vi "数据模拟实测.vi"() -> ()   [LabVIEW 2020]
uses:
  <vilib>/Utility/error.llb/DialogType.ctl
  <vilib>/Analysis/baseanly.llb/Mean (DBL).vi
  <vilib>/Utility/inputDevices.llb/mouseAcquire.vi
  GlobalVariable.vi
  <vilib>/Analysis/NI_AALBase.lvlib
panel:
  in  "退出":bool
  in  "选项卡控件":enum32{"数据文件界面", "实时模拟界面"}(tab)
  out "历史波形图":dbl[][](graph)
  out "数据采集起止时间":string
  in  "曲线标尺":bool[](array[boolean])=[TRUE, TRUE, TRUE, TRUE, TRUE, TRUE, TRUE, TRUE]
  in  "曲线隐显":bool[](array[boolean])=[TRUE, TRUE, TRUE, TRUE, TRUE, TRUE, TRUE, TRUE]
  in  "开始模拟":bool
  in  "重选文件":bool
  in  "刻棒选择":u16(ring) items=["D棒位"]
  in  "因子选择":i32(ring) items=["C1", "C2", "C3", "C4", "C5", "C6", "C7", "C8", "C9", "10"]
  in  "上段信号选择":i32(ring) items=["电流1", "电流2"]
  in  "下段信号选择":u16(ring)=1 items=["电流1", "电流2"]
  out "实时波形图":sgl[][](graph) caption="Waveform Chart - Dark"
  in  "曲线开关0":bool
  in  "曲线开关1":bool
  in  "曲线开关2":bool
  in  "曲线开关3":bool
  in  "曲线开关5":bool
  in  "曲线开关4":bool
  in  "自动调整Y标尺？":bool
  in  "自动/手动调整X标尺？":bool
  out "曲线0数字":dbl caption="电流1"
  out "曲线1数字":dbl caption="电流1反应性"
  out "曲线2数字":dbl caption="电流2"
  out "曲线3数字":dbl caption="电流2反应性"
  out "曲线4数字":dbl caption="D棒位"
  out "曲线5数字":dbl
  in  "仿真加速或减速倍数":dbl(slide)=0.1 min=-5.0 max=10.0 step=0.1 scale=-5.0..10.0 scale format="%#.1f"
  in  "备注说明":string
  out "上下段比值":dbl format="%0.2f"
  in  "合并DSF":bool
  in  "DRWM启用":bool
  in  "上段本底":dbl
  in  "下段本底":dbl
  in  "X标尺最小+":bool
  in  "X标尺最小-":bool
  in  "Y标尺最小+":bool
  in  "Y标尺最小-":bool
  in  "Y标尺最大+":bool
  in  "Y标尺最大-":bool
  out "AllStop":bool
  # "DRWM选项"
  # "DRWM控制"
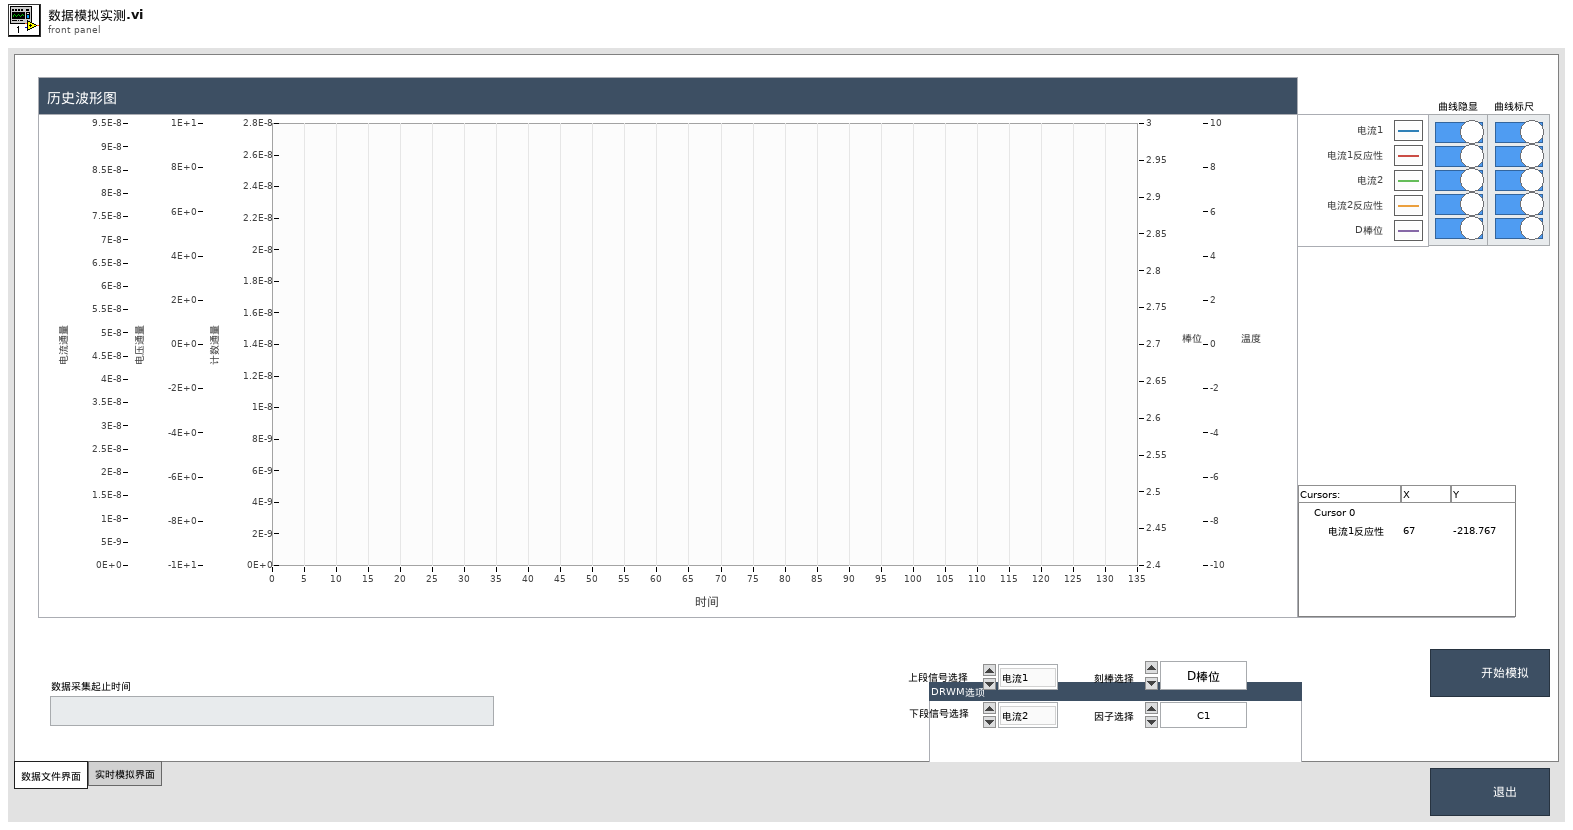
[diagram p1: front panel]
types:
  T1 = enum32{"Page Enabled", "Page Disabled", "Page Disabled & Grayed"}
  T2 = enum8{"Enabled", "Disabled", "Disabled and Grayed Out"}
  T3 = enum16{"open", "open or create", "create or replace", "create", "open (read only)"}
  T4 = typedef "DialogType.ctl" = u16
  T5 = cluster{"button 1":bool, "button 2":bool, "button 3":bool, "button 4":bool}
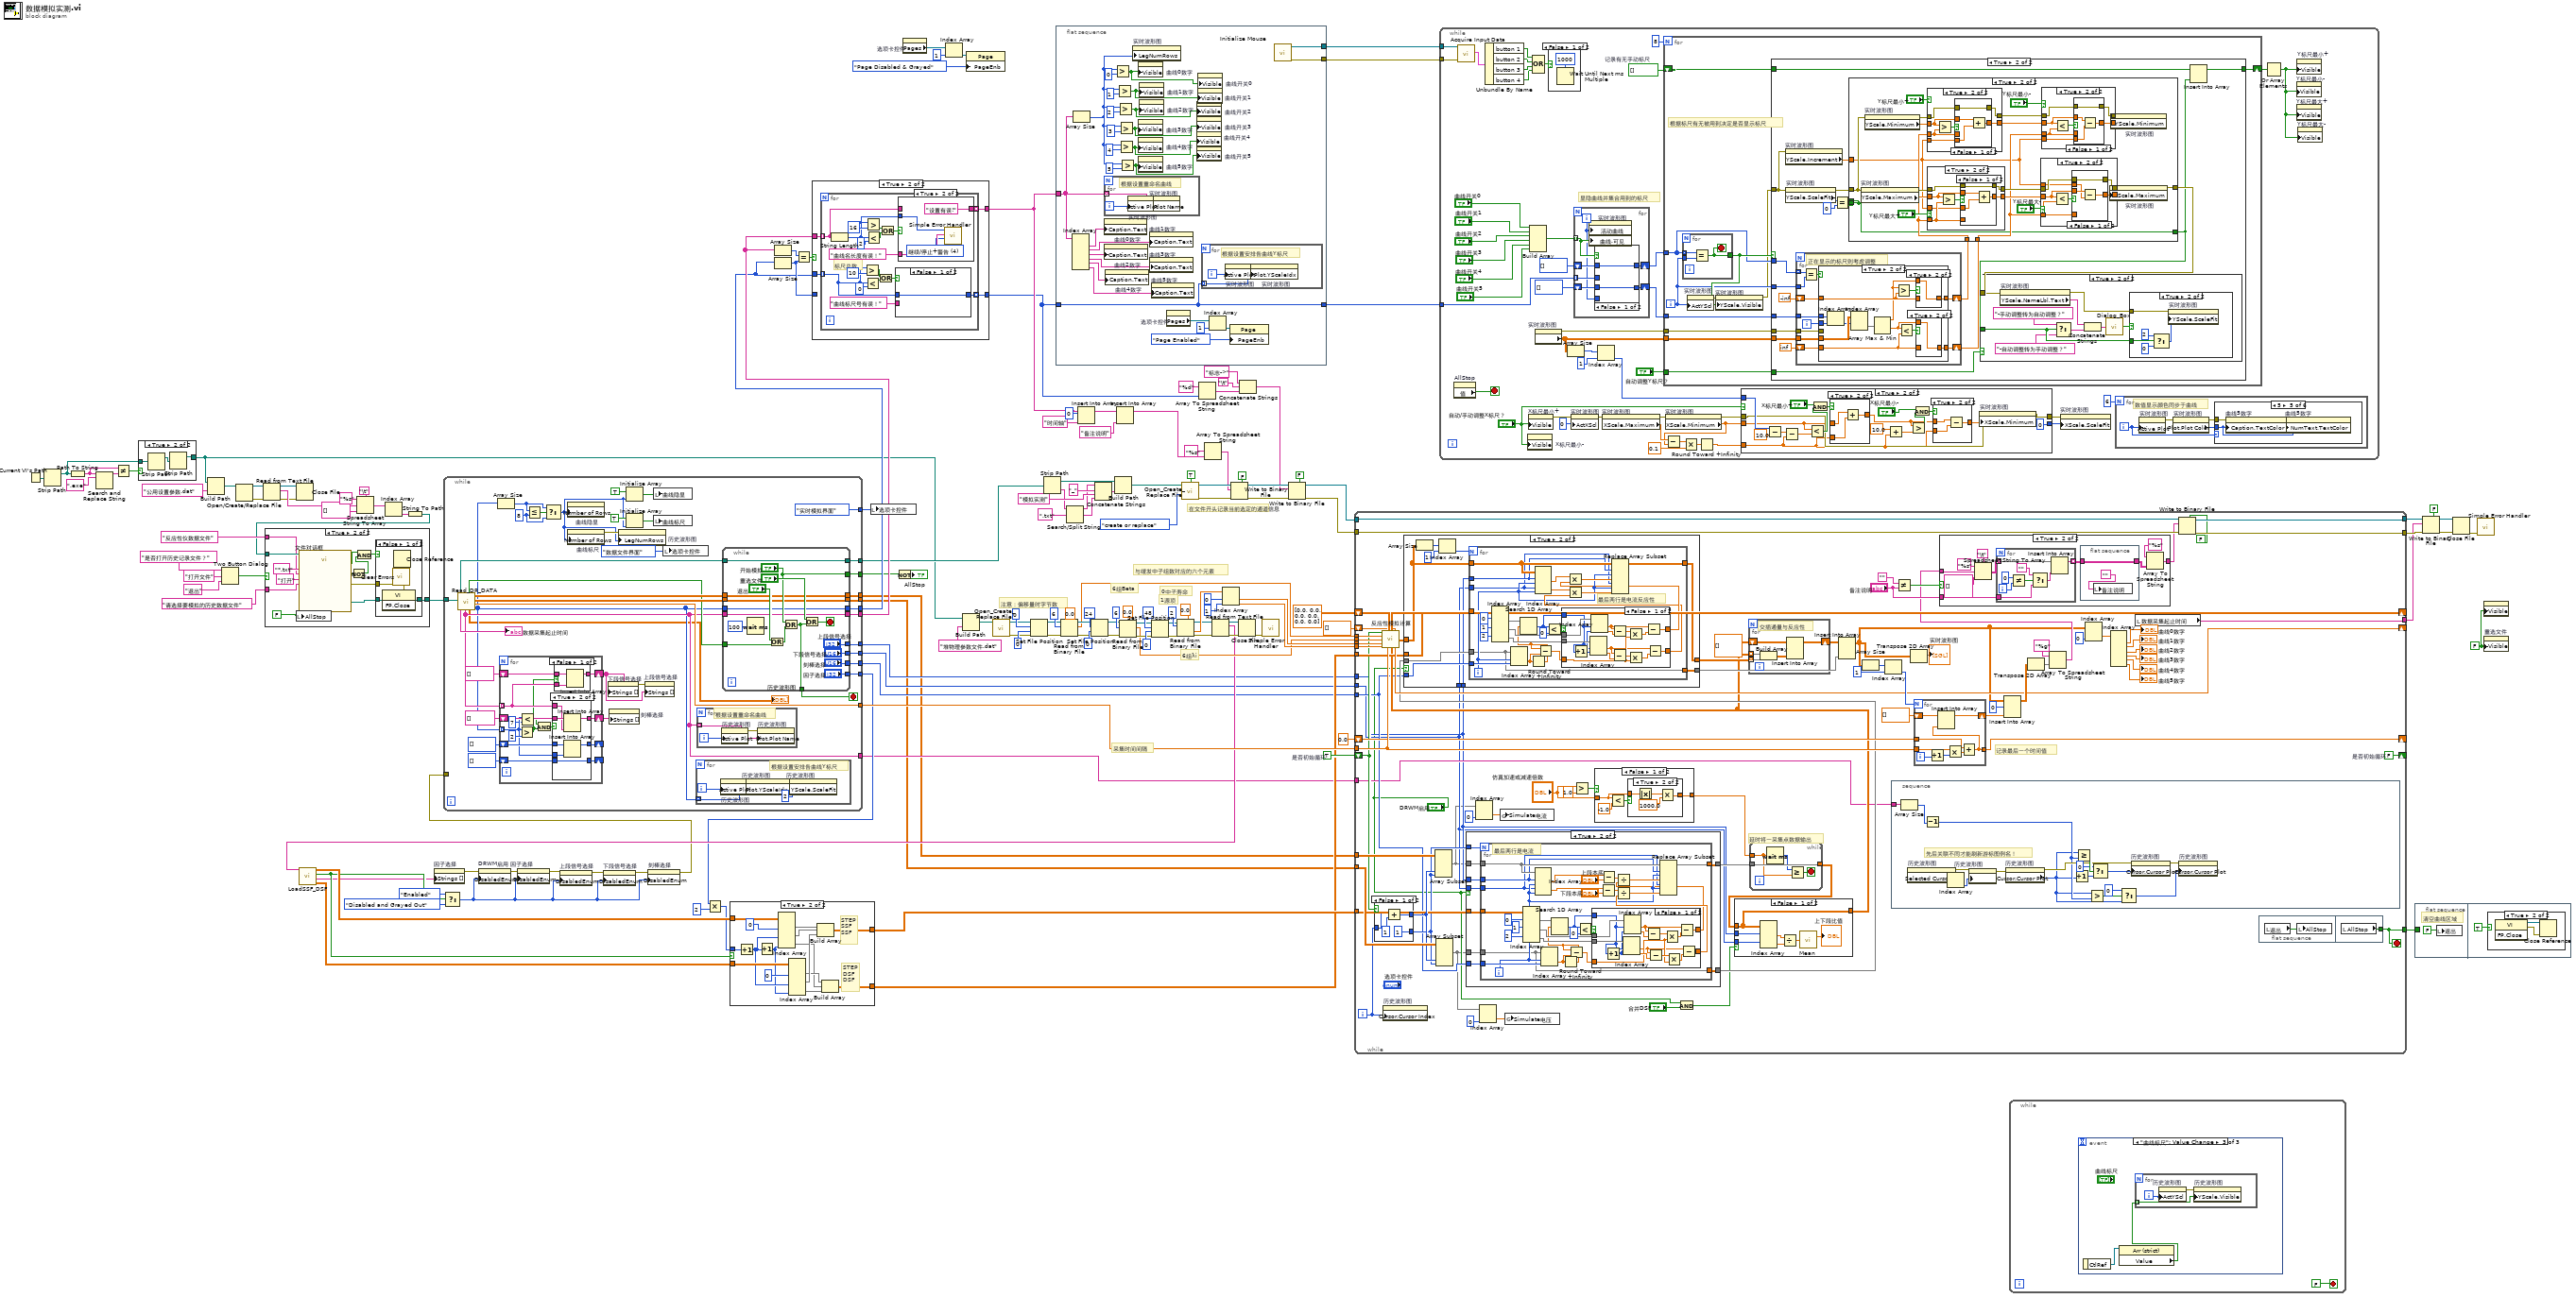
[diagram p0: block diagram]
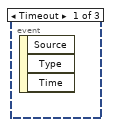
[diagram p2: hidden frame]
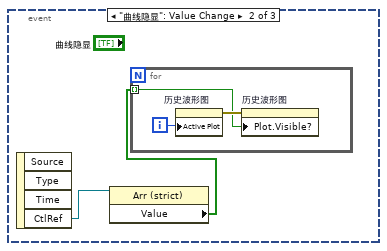
[diagram p3: hidden frame]
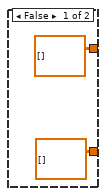
[diagram p4: hidden frame]
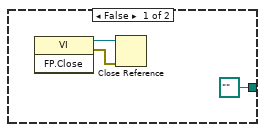
[diagram p5: hidden frame]
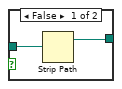
[diagram p7: hidden frame]
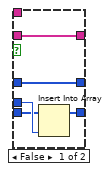
[diagram p9: hidden frame]
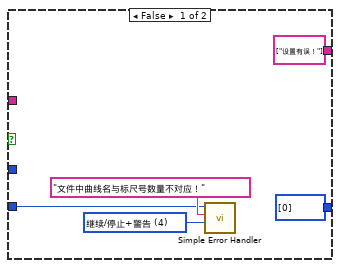
[diagram p11: hidden frame]
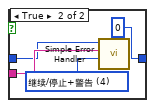
[diagram p12: hidden frame]
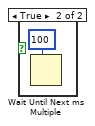
[diagram p14: hidden frame]
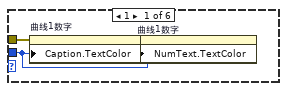
[diagram p15: hidden frame]
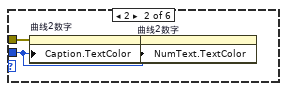
[diagram p16: hidden frame]
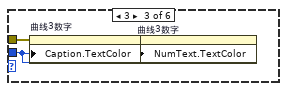
[diagram p17: hidden frame]
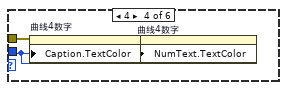
[diagram p18: hidden frame]
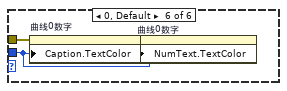
[diagram p19: hidden frame]
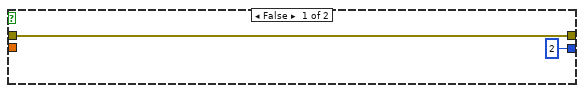
[diagram p20: hidden frame]
diagram:
  w5 = FALSE ("Visible")
  w122 = TRUE  # 是否初始循环
  # "6组λi"
  # "在文件开头记录当前选定的通道信息"
  # "采集时间间隔"
  # "注意：偏移量时字节数"
  # "与缓发中子组数对应的六个元素"
  # "0中子寿命"
  # "1源项"
  # "6组Beta"
  n1 = Current VI's Path() -> (path=w66:path)
  n2 = Strip Path(path=w66) -> (stripped path=w61:path)  [unwired: 1 out]
  n3 = Path To String(path=w61) -> (string=w63:string)
  n4 = Search and Replace String(input string=w63, search string=".exe" ("搜索字符串")) -> (result string=w64:string)  [unwired: 6 in, 3 out]
  n5 = Not Equal?(x=w63, y=w64) -> (x != y?=w62:bool)
  n6 = case shown="True" w62 {
    tunnel: w61 -> [w155 w158]
    tunnel: [w154 w156] -> w29
    frame False {
      n7 = Strip Path(path=w155) -> (stripped path=w154:path)  [unwired: 1 out]
    }
    frame True {
      n8 = Strip Path(path=w158) -> (stripped path=w157:path)  [unwired: 1 out]
      n9 = Strip Path(path=w157) -> (stripped path=w156:path)  [unwired: 1 out]
    }
  }
  n10 = Build Path(base path=w29, name or relative path="公用设置参数.dat") -> (appended path=w47:path)
  n11 = Two Button Dialog(message="是否打开历史记录文件？", 1:"退出" ("message"), 2:"打开文件" ("message")) -> (T button?=w57:bool)
  n12 = Open/Create/Replace File(file path (use dialog)=w47) -> (refnum out=w50:refnum<file>, error out=w51:errorcluster)  [unwired: 5 in, 1 out]
  n13 = Read from Text File(file (use dialog)=w50, error in=w51) -> (refnum out=w49:refnum<file>, text=w55:string, error out=w48:errorcluster)  [unwired: 1 in, 2 out]
  n14 = Close File(refnum=w49, error in=w48) -> ()  [unwired: 2 out]
  n15 = Spreadsheet String To Array(delimiter (Tab)="\t", format string="%s", spreadsheet string=w55, array type (2D Dbl)=string[] [] ("添加的数组")) -> (array=w56:string[])
  n16 = Index Array(array=w56) -> (element=w45:string)  [unwired: 1 in]
  n17 = String To Path(string=w45) -> (path=w58:path)
  n18 = case shown="True" w57 {
    tunnel: w58 -> [_ w174]
    tunnel: "请选择要模拟的历史数据文件" ("prompt") -> [_ w170]
    tunnel: "反应性仪数据文件" ("pattern label") -> [_ w169]
    tunnel: [path "" ("selected path") w167] -> w41
    frame False {
      n19 = invoke class="VI" method="FP.Close"() -> (reference out=w160:refnum<vi>, error out=w159:errorcluster)  [unwired: 3 in, 1 out]
      n20 = Close Reference(reference=w160, error in (no error)=w159) -> ()  [unwired: 1 out]
    }
    frame True {
      n21 = local write "AllStop"(FALSE ("退出程序")) -> ()
      n22 = call "文件对话框"("start path"=w174, "prompt"=w170, "button label"="打开", "pattern (all files)"="*.txt", "pattern label"=w169) -> ("selected path"=w168:path, "exists"=w165:bool, "cancelled"=w166:bool, "error out"=w162:errorcluster)  [unwired: 7 in]
      n23 = Not(x=w166) -> (.not. x?=w164:bool)
      n24 = And(x=w165, y=w164) -> (x .and. y?=w163:bool)
      n25 = case shown="False" w163 {
        tunnel: w168 -> [w178 w179]
        tunnel: [w178 w179] -> w167
        tunnel: w162 -> [w177 _]
        frame False {
          n26 = invoke class="VI" method="FP.Close"() -> (reference out=w175:refnum<vi>, error out=w176:errorcluster)  [unwired: 3 in, 1 out]
          n27 = call <vilib>:"Clear Errors.vi"("error in (no error)"=w177) -> ()  [unwired: 5 in, 2 out]
          n28 = Close Reference(reference=w175, error in (no error)=w176) -> ()  [unwired: 1 out]
        }
        frame True {
        }
      }
    }
  }
  n29 = property on="选项卡控件" class="TabCtl (strict)"() -> ("Pages"=w1:refnum<vi>[])  [unwired: 2 in, 2 out]
  n30 = Index Array(array=w1, index=1) -> (element=w2:refnum<vi>)
  n31 = Build Path(base path=w29, name or relative path="堆物理参数文件.dat" ("string")) -> (appended path=w134:path)
  n32 = property class="Page"(reference=w2, "PageEnb"=T1."Page Disabled & Grayed" ("Page Enabled State")) -> ()  [unwired: 1 in, 2 out]
  n33 = call <vilib>:"Open_Create_Replace File.vi"("file path"=w134) -> ("error out"=w118:errorcluster, "refnum"=w119:refnum<file>)  [unwired: 7 in, 2 out]
  n34 = Set File Position(offset (in bytes) (0)=0, refnum=w119, from (0:start)=0, error in=w118) -> (refnum out=w131:refnum<file>, error out=w130:errorcluster)
  n35 = flat-sequence {
    tunnel: w85 -> [w194]
    tunnel: [w184] -> w112
    tunnel: w84 -> [w184]
    tunnel: [w186] -> w121
    tunnel: [w185] -> w120
    frame #0 {
      n36 = Index Array(array=w194) -> (element #1=w206:string, element #2=w205:string, element #3=w204:string, element #4=w203:string, element #5=w202:string, element #6=w201:string)  [unwired: 6 in]
      n37 = Array Size(array=w194) -> (size(s)=w187:i32)
      n38 = property on="曲线0数字" class="DigNum (strict)"("Caption.Text"=w206) -> ()  [unwired: 2 in, 2 out]
      n39 = for {
        tunnel: w194 -> [w211] mode=indexing
        i -> [w212]
        # "根据设置重命名曲线"
        n40 = property on="实时波形图" class="WFChart (strict)"("Active Plot"=w212) -> (error out=w210:errorcluster)  [unwired: 2 in, 1 out]
        n41 = property on="实时波形图" class="WFChart (strict)"(error in=w210, "Plot.Plot Name"=w211) -> ()  [unwired: 1 in, 2 out]
      }
      n42 = property on="曲线2数字" class="DigNum (strict)"("Caption.Text"=w204) -> ()  [unwired: 2 in, 2 out]
      n43 = property on="曲线4数字" class="DigNum (strict)"("Caption.Text"=w202) -> ()  [unwired: 2 in, 2 out]
      n44 = Greater?(x=w187, y=0) -> (0:w193:bool)
      n45 = Greater?(x=w187, y=1) -> (0:w192:bool)
      n46 = Greater?(x=w187, y=2) -> (0:w191:bool)
      n47 = Greater?(x=w187, y=3) -> (0:w190:bool)
      n48 = Greater?(x=w187, y=4) -> (0:w189:bool)
      n49 = Greater?(x=w187, y=5) -> (0:w188:bool)
      n50 = property on="实时波形图" class="WFChart (strict)"("LegNumRows"=w187) -> ()  [unwired: 2 in, 2 out]
      n51 = property on="曲线0数字" class="DigNum (strict)"("Visible"=w193) -> ()  [unwired: 2 in, 2 out]
      n52 = property on="曲线3数字" class="DigNum (strict)"("Visible"=w190) -> ()  [unwired: 2 in, 2 out]
      n53 = property on="曲线4数字" class="DigNum (strict)"("Visible"=w189) -> ()  [unwired: 2 in, 2 out]
      n54 = property on="曲线5数字" class="DigNum (strict)"("Visible"=w188) -> ()  [unwired: 2 in, 2 out]
      n55 = property on="曲线1数字" class="DigNum (strict)"("Visible"=w192) -> ()  [unwired: 2 in, 2 out]
      n56 = property on="曲线2数字" class="DigNum (strict)"("Visible"=w191) -> ()  [unwired: 2 in, 2 out]
      n57 = property on="曲线1数字" class="DigNum (strict)"("Caption.Text"=w205) -> ()  [unwired: 2 in, 2 out]
      n58 = property on="曲线3数字" class="DigNum (strict)"("Caption.Text"=w203) -> ()  [unwired: 2 in, 2 out]
      n59 = property on="曲线5数字" class="DigNum (strict)"("Caption.Text"=w201) -> ()  [unwired: 2 in, 2 out]
      n60 = property on="选项卡控件" class="TabCtl (strict)"() -> ("Pages"=w183:refnum<vi>[])  [unwired: 2 in, 2 out]
      n61 = property on="曲线开关4" class="Bool (strict)"("Visible"=w189) -> ()  [unwired: 2 in, 2 out]
      n62 = property on="曲线开关2" class="Bool (strict)"("Visible"=w191) -> ()  [unwired: 2 in, 2 out]
      n63 = property on="曲线开关3" class="Bool (strict)"("Visible"=w190) -> ()  [unwired: 2 in, 2 out]
      n64 = property on="曲线开关5" class="Bool (strict)"("Visible"=w188) -> ()  [unwired: 2 in, 2 out]
      n65 = property on="曲线开关1" class="Bool (strict)"("Visible"=w192) -> ()  [unwired: 2 in, 2 out]
      n66 = property on="曲线开关0" class="Bool (strict)"("Visible"=w193) -> ()  [unwired: 2 in, 2 out]
      n67 = for {
        tunnel: w184 -> [w207] mode=indexing
        i -> [w209]
        # "根据设置安排各曲线Y标尺"
        n68 = property on="实时波形图" class="WFChart (strict)"("Active Plot"=w209) -> (error out=w208:errorcluster)  [unwired: 2 in, 1 out]
        n69 = property on="实时波形图" class="WFChart (strict)"(error in=w208, "Plot.YScaleIdx"=w207) -> ()  [unwired: 1 in, 2 out]
      }
      n70 = Index Array(array=w183, index=1) -> (element=w182:refnum<vi>)
      n71 = property class="Page"(reference=w182, "PageEnb"=T1."Page Enabled" ("Page Enabled State")) -> ()  [unwired: 1 in, 2 out]
      n72 = call <vilib>:"Initialize Mouse.vi"() -> ("error out"=w186:errorcluster, "device ID"=w185:refnum<k1>)  [unwired: 1 in, 9 out]
    }
  }
  n73 = Read from Binary File(5:sgl 0.0, 8:w130, 10:6, 11:w131) -> (0:w126:errorcluster, 2:w117:sgl[], 3:w127:refnum<file>)  [unwired: 2 in, 1 out]
  n74 = Set File Position(offset (in bytes) (0)=24, refnum=w127, from (0:start)=0, error in=w126) -> (refnum out=w129:refnum<file>, error out=w128:errorcluster)
  n75 = Read from Binary File(5:sgl 0.0, 8:w128, 10:6, 11:w129) -> (0:w124:errorcluster, 2:w75:sgl[], 3:w125:refnum<file>)  [unwired: 2 in, 1 out]
  n76 = Set File Position(offset (in bytes) (0)=48, refnum=w125, from (0:start)=0, error in=w124) -> (refnum out=w133:refnum<file>, error out=w132:errorcluster)
  n77 = Read from Binary File(5:sgl 0.0, 8:w132, 10:2, 11:w133) -> (0:w39:errorcluster, 2:w144:sgl[], 3:w40:refnum<file>)  [unwired: 2 in, 1 out]
  n78 = Read from Text File(file (use dialog)=w40, error in=w39) -> (refnum out=w38:refnum<file>, text=w36:string, error out=w37:errorcluster)  [unwired: 1 in, 2 out]
  n79 = call "LoadSSF_DSF.vi"("SF_PATH"=w36) -> ("下段因子数据"=w34:dbl[][], "因子棒号"=w25:string[], "SF_OK"=w28:bool, "上段因子数据"=w35:dbl[][])  [unwired: 6 in, 1 out]
  n80 = property on="因子选择" class="Ring (strict)"("Strings []"=w25) -> (error out=w24:errorcluster)  [unwired: 2 in, 1 out]
  n81 = Select(t=T2."Enabled" ("禁用"), s=w28, f=T2."Disabled and Grayed Out" ("禁用")) -> (s? t:f=w19:T2)
  n82 = property on="DRWM启用" class="Bool (strict)"(error in=w24, "DisabledEnum"=w19) -> (error out=w23:errorcluster)  [unwired: 1 in, 1 out]
  n83 = property on="因子选择" class="Ring (strict)"(error in=w23, "DisabledEnum"=w19) -> (error out=w21:errorcluster)  [unwired: 1 in, 1 out]
  n84 = property on="上段信号选择" class="Ring (strict)"(error in=w21, "DisabledEnum"=w19) -> (error out=w20:errorcluster)  [unwired: 1 in, 1 out]
  n85 = property on="下段信号选择" class="Ring (strict)"(error in=w20, "DisabledEnum"=w19) -> (error out=w18:errorcluster)  [unwired: 1 in, 1 out]
  n86 = property on="刻棒选择" class="Ring (strict)"(error in=w18, "DisabledEnum"=w19) -> (error out=w17:errorcluster)  [unwired: 1 in, 1 out]
  n87 = while {
    tunnel: [w249] -> w11
    tunnel: [w251] -> w69
    tunnel: [w250] -> w111
    tunnel: [w247] -> w110
    tunnel: [w248] -> w10
    tunnel: [w240] -> w108
    tunnel: [w245] -> w68
    tunnel: w41 -> [w244]
    tunnel: w17 -> [_]
    tunnel: [w237] -> w22
    tunnel: [w229] -> w14
    tunnel: [w228] -> w15
    tunnel: [w227] -> w16
    tunnel: [w226] -> w13
    tunnel: [enum32{"数据文件界面", "实时模拟界面"}."实时模拟界面" ("选项卡控件")] -> w12
    stop <- w246 stop-if-true
    w224 = 8 ("y")
    n88 = call "Read_DR_DATA.vi"("文件路径"=w244) -> ("标尺号"=w222:i32[], "时间步长"=w240:dbl, "P2数据"=w242:dbl[][], "通量数据"=w243:dbl[][], "曲线数据"=→"历史波形图":dbl[][], "读取正确?"=w241:bool, "曲线名称"=w226:string[], "数据采集起止时间"=→"数据采集起止时间":string, "filepath"=w239:path)  [unwired: 2 in]
    n89 = Array Size(array=w222) -> (size(s)=w223:i32)
    n90 = for {
      tunnel: w226 -> [w253] mode=indexing
      tunnel: w222 -> [w259] mode=indexing
      shift-right: [w265] -> w230
      shift-left: string[] [] -> [w266]
      shift-right: [w263] -> _
      shift-left: i32[] [] ("标尺号") -> [w264]
      shift-right: [w254] -> w231
      shift-left: string[] [] -> [w255]
      shift-right: [w261] -> _
      shift-left: i32[] [] ("标尺号") -> [w262]
      n91 = Greater?(x=w259, y=2) -> (0:w252:bool)
      n92 = Less?(x=w259, y=7) -> (x < y?=w257:bool)
      n93 = And(x=w257, y=w252) -> (x .and. y?=w256:bool)
      n94 = case shown="True" w256 {
        tunnel: w266 -> [w275 w282]
        tunnel: [w275 w281] -> w265
        tunnel: w264 -> [w274 w280]
        tunnel: [w274 w279] -> w263
        tunnel: w259 -> [w273 w278]
        tunnel: w253 -> [_ w277]
        tunnel: w262 -> [w272 w276]
        tunnel: [w271 w276] -> w261
        frame False {
          n95 = Insert Into Array(array=w272, new element=w273) -> (w271:i32[])  [unwired: 1 in]
        }
        frame True {
          n96 = Insert Into Array(array=w282, new element=w277) -> (w281:string[])  [unwired: 1 in]
          n97 = Insert Into Array(array=w280, new element=w278) -> (w279:i32[])  [unwired: 1 in]
        }
      }
      n98 = case shown="False" w252 {
        tunnel: w255 -> [w269 w270]
        tunnel: [w268 w270] -> w254
        tunnel: w253 -> [w267 _]
        frame False {
          n99 = Insert Into Array(array=w269, new element=w267) -> (w268:string[])  [unwired: 1 in]
        }
        frame True {
        }
      }
    }
    n100 = Less Or Equal?(x=w223, y=w224) -> (x <= y?=w225:bool)
    n101 = Select(t=w223, s=w225, f=w224) -> (s? t:f=w215:i32)
    n102 = property on="曲线隐显" class="Arr (strict)"("Number of Rows"=w215) -> ()  [unwired: 2 in, 2 out]
    n103 = property on="曲线标尺" class="Arr (strict)"("Number of Rows"=w215) -> (error out=w216:errorcluster)  [unwired: 2 in, 1 out]
    n104 = property on="下段信号选择" class="Ring (strict)"("Strings []"=w231) -> (error out=w232:errorcluster)  [unwired: 2 in, 1 out]
    n105 = property on="刻棒选择" class="Ring (strict)"("Strings []"=w230) -> ()  [unwired: 2 in, 2 out]
    n106 = property on="历史波形图" class="WFGraph (strict)"(error in=w216, "LegNumRows"=w215) -> ()  [unwired: 1 in, 2 out]
    n107 = Initialize Array(TRUE ("开始模拟"), w215) -> (w219:bool[])
    n108 = Initialize Array(TRUE ("开始模拟"), w215) -> (w218:bool[])
    n109 = property on="上段信号选择" class="Ring (strict)"(error in=w232, "Strings []"=w231) -> ()  [unwired: 1 in, 2 out]
    n110 = local write "曲线隐显"(w219) -> ()
    n111 = local write "曲线标尺"(w218) -> ()
    n112 = local write "选项卡控件"(enum32{"数据文件界面", "实时模拟界面"}."数据文件界面" ("选项卡控件")) -> ()
    n113 = for {
      tunnel: w222 -> [w285] mode=indexing
      i -> [w287]
      # "根据设置安排各曲线Y标尺"
      n114 = property on="历史波形图" class="WFGraph (strict)"("Active Plot"=w287) -> (error out=w286:errorcluster)  [unwired: 2 in, 1 out]
      n115 = property on="历史波形图" class="WFGraph (strict)"(error in=w286, "Plot.YScaleIdx"=w285) -> (error out=w284:errorcluster)  [unwired: 1 in, 1 out]
      n116 = property on="历史波形图" class="WFGraph (strict)"(error in=w284, "YScale.ScaleFit"=u8 2 ("Y标尺.标尺调节")) -> ()  [unwired: 1 in, 2 out]
    }
    n117 = for {
      tunnel: w226 -> [w289] mode=indexing
      i -> [w290]
      # "根据设置重命名曲线"
      n118 = property on="历史波形图" class="WFGraph (strict)"("Active Plot"=w290) -> (error out=w288:errorcluster)  [unwired: 2 in, 1 out]
      n119 = property on="历史波形图" class="WFGraph (strict)"(error in=w288, "Plot.Plot Name"=w289) -> ()  [unwired: 1 in, 2 out]
    }
    n120 = while {
      tunnel: [w299] -> w249
      tunnel: [w297] -> w250
      tunnel: w242 -> [w299]
      tunnel: w226 -> [w297]
      tunnel: [w305] -> w246
      tunnel: ["开始模拟"] -> w251
      tunnel: w241 -> [w302]
      tunnel: w243 -> [w300]
      tunnel: [w300] -> w248
      tunnel: w222 -> [w298]
      tunnel: [w298] -> w247
      tunnel: [w295] -> w245
      tunnel: w239 -> [w295]
      tunnel: ["因子选择"] -> w237
      tunnel: ["上段信号选择"] -> w229
      tunnel: ["下段信号选择"] -> w228
      tunnel: ["刻棒选择"] -> w227
      stop <- w296 stop-if-true
      n121 = Wait (ms)(milliseconds to wait=u32 100 ("等待时间（毫秒）")) -> ()  [unwired: 1 out]
      n122 = Or(x="退出", y=w302) -> (x .or. y?=w303:bool)
      n123 = Or(x="开始模拟", y=w303) -> (x .or. y?=w305:bool)
      n124 = Or(x="重选文件", y=w305) -> (x .or. y?=w296:bool)
    }
  }
  n125 = Multiply(x=w22, y=u16 2) -> (x*y=w32:i32)
  n126 = case shown="True" w28 {
    tunnel: w35 -> [_ w324]
    tunnel: w34 -> [_ w322]
    tunnel: w32 -> [_ w323]
    tunnel: [dbl[][] [] w315] -> w31
    tunnel: [dbl[][] [] w314] -> w30
    frame False {
    }
    frame True {
      # "STEP\nDSF\nDSF"
      # "STEP\nSSF\nSSF"
      n127 = Increment(x=w323) -> (x+1=w311:i32)
      n128 = Increment(x=w311) -> (x+1=w310:i32)
      n129 = Index Array(array=w324, index (col) #1=0 ("索引 (行)"), index (col) #2=w311, index (col) #3=w310) -> (element #1=w321:dbl[], element #2=w320:dbl[], element #3=w317:dbl[])  [unwired: 3 in]
      n130 = Index Array(array=w322, index (col) #1=0 ("索引 (行)"), index (col) #2=w311, index (col) #3=w310) -> (element #1=w318:dbl[], element #2=w319:dbl[], element #3=w316:dbl[])  [unwired: 3 in]
      n131 = Build Array(w321, w320, w319) -> (w315:dbl[][])
      n132 = Build Array(w318, w317, w316) -> (w314:dbl[][])
    }
  }
  n133 = Array Size(array=w111) -> (size(s)=w116:i32)
  n134 = Array Size(array=w110) -> (size(s)=w114:i32)
  n135 = Equal?(x=w116, y=w114) -> (x = y?=w115:bool)
  n136 = case shown="True" w115 {
    tunnel: w114 -> [w327 _]
    tunnel: w110 -> [_ w333]
    tunnel: w111 -> [_ w332]
    tunnel: [i32[] [0] w331] -> w84
    tunnel: [string[] ["设置有误！"] w330] -> w85
    frame False {
      w329 = T4 4 items=["无对话框", "确定信息", "继续或停止信息", "确定信息＋警告", "继续/停止+警告"] ("type of dialog (OK msg:1)")
      n137 = call <vilib>:"Simple Error Handler.vi"("error code (no error:0)"=w327, "error source (\" \")"="文件中曲线名与标尺号数量不对应！" ("error source (\" \")"), "type of dialog (OK msg:1)"=w329) -> ()  [unwired: 2 in, 5 out]
    }
    frame True {
      n138 = for {
        tunnel: w333 -> [w338] mode=indexing
        tunnel: w332 -> [w335] mode=indexing
        tunnel: [w336] -> w331 mode=indexing
        tunnel: [w334] -> w330 mode=indexing
        # "标尺总数"
        n139 = String Length(string=w335) -> (length=w340:i32)
        n140 = Greater?(x=w338, y=10) -> (0:w343:bool)
        n141 = Less?(x=w338, y=0) -> (x < y?=w342:bool)
        n142 = Greater?(x=w340, y=16) -> (0:w347:bool)
        n143 = Less?(x=w340, y=2) -> (x < y?=w348:bool)
        n144 = Or(x=w343, y=w342) -> (x .or. y?=w339:bool)
        n145 = Or(x=w347, y=w348) -> (x .or. y?=w346:bool)
        n146 = case shown="False" w339 {
          tunnel: "曲线标尺号有误！" ("error source (\" \")") -> [_ w355]
          tunnel: w338 -> [w351 w354]
          tunnel: [w351 0] -> w336
          frame False {
          }
          frame True {
            w353 = T4 4 items=["无对话框", "确定信息", "继续或停止信息", "确定信息＋警告", "继续/停止+警告"] ("type of dialog (OK msg:1)")
            n147 = call <vilib>:"Simple Error Handler.vi"("error code (no error:0)"=w354, "error source (\" \")"=w355, "type of dialog (OK msg:1)"=w353) -> ()  [unwired: 2 in, 5 out]
          }
        }
        n148 = case shown="True" w346 {
          tunnel: "曲线名长度有误！" ("error source (\" \")") -> [_ w360]
          tunnel: w340 -> [_ w359]
          tunnel: w335 -> [w356 _]
          tunnel: [w356 "设置有误!"] -> w334
          frame False {
          }
          frame True {
            w358 = T4 4 items=["无对话框", "确定信息", "继续或停止信息", "确定信息＋警告", "继续/停止+警告"] ("type of dialog (OK msg:1)")
            n149 = call <vilib>:"Simple Error Handler.vi"("error code (no error:0)"=w359, "error source (\" \")"=w360, "type of dialog (OK msg:1)"=w358) -> ()  [unwired: 2 in, 5 out]
          }
        }
      }
    }
  }
  n150 = local write "选项卡控件"(w12) -> ()
  n151 = Not(x=w69) -> (.not. x?=→"AllStop":bool)
  n152 = Strip Path(path=w68) -> (stripped path=w70:path, name=w9:string)
  n153 = Search/Split String(string=w9, search string/char (-)=".txt" ("搜索字符串/字符(-)")) -> (substring before match=w7:string, match + rest of string=w6:string)  [unwired: 1 in, 1 out]
  n154 = Insert Into Array(array=w85, index=0 ("索引"), new element="时间轴" ("新元素/子数组")) -> (w90:string[])
  n155 = Concatenate Strings ("连接字符串")(w7, "_" ("string"), "模拟实测" ("字符串"), w6) -> (w71:string)
  n156 = Build Path(base path=w70, name or relative path=w71) -> (appended path=w72:path)
  n157 = Insert Into Array(array=w90, new element="备注说明" ("新元素/子数组")) -> (w89:string[])  [unwired: 1 in]
  n158 = call <vilib>:"Open_Create_Replace File.vi"("advisory dialog? (display:T)"=TRUE, "function (open:0)"=T3."create or replace", "file path"=w72) -> ("error out"=w106:errorcluster, "refnum"=w103:refnum<file>)  [unwired: 5 in, 2 out]
  n159 = Array To Spreadsheet String(array=w84, 3:"%d" ("format string")) -> (spreadsheet string=w94:string)  [unwired: 1 in]
  n160 = Array To Spreadsheet String(array=w89, 3:"%s" ("format string")) -> (spreadsheet string=w101:string)  [unwired: 1 in]
  n161 = Index Array(array=w144, index #1=0, index #2=1) -> (element #1=w137:sgl, element #2=w136:sgl)
  n162 = Write to Binary File(file (use dialog)=w103, data=w101, error in=w106, 5:FALSE ("预置数组或字符串大小？(T)")) -> (refnum out=w96:refnum<file>, error out=w95:errorcluster)  [unwired: 2 in, 1 out]
  n163 = Close File(refnum=w38, error in=w37) -> (error out=w123:errorcluster)  [unwired: 1 out]
  n164 = Concatenate Strings("标志->" ("字符串"), "\t", w94) -> (w91:string)
  n165 = call <vilib>:"Simple Error Handler.vi"("error in (no error)"=w123) -> ()  [unwired: 4 in, 5 out]
  n166 = Write to Binary File(file (use dialog)=w96, data=w91, error in=w95, 5:FALSE ("预置数组或字符串大小？(T)")) -> (refnum out=w86:refnum<file>, error out=w87:errorcluster)  [unwired: 2 in, 1 out]
  n167 = while {
    shift-right: [w430] -> _
    shift-left: sgl[][] [[0.0], [0.0], [0.0], [0.0], [0.0], [0.0]] -> [w431]
    tunnel: w117 -> [w432]
    tunnel: w75 -> [w437]
    tunnel: w137 -> [w429]
    tunnel: w136 -> [w428]
    shift-right: [w436] -> _
    shift-left: w122 -> [w377]
    tunnel: w86 -> [w427]
    tunnel: w87 -> [w435]
    tunnel: [w361] -> w113
    tunnel: [w434] -> w79
    tunnel: w108 -> [w398]
    tunnel: [w426] -> w80
    tunnel: w10 -> [w410]
    tunnel: w11 -> [w409]
    tunnel: [w390] -> w74
    shift-right: [w395] -> _
    shift-left: 0.0 -> [w394]
    shift-right: [w391] -> _
    shift-left: sgl[] [] ("N(0)OUT") -> [w392]
    tunnel: w31 -> [w386]
    tunnel: w30 -> [w385]
    tunnel: w16 -> [w376]
    tunnel: w15 -> [w373]
    tunnel: w14 -> [w374]
    tunnel: w13 -> [w375]
    i -> [w378]
    stop <- w361 stop-if-true
    w436 = FALSE  # 是否初始循环
    # "记录最后一个时间值"
    # "延时将一采集点数据输出"
    n168 = case shown="False" w377 {
      tunnel: [w622 0 ("索引")] -> w407
      tunnel: [1 ("索引") 2 ("索引")] -> w383
      tunnel: w378 -> [w621 _]
      frame False {
        n169 = Add(x=w621, y=1) -> (x+y=w622:i32)
      }
      frame True {
      }
    }
    n170 = property on="历史波形图" class="WFGraph (strict)"("Cursor.Cursor Index"=w378) -> ()  [unwired: 2 in, 2 out]
    n171 = Array Subset(array=w410, index (col)=w407, length (col)=w383) -> (w369:dbl[][])  [unwired: 2 in]
    n172 = Array Subset(array=w409, index (col)=w407, length (col)=w383) -> (w368:dbl[][])  [unwired: 2 in]
    n173 = case shown="True" "DRWM启用" {
      tunnel: w369 -> [w530 w537]
      tunnel: [w530 w536] -> w389
      tunnel: w368 -> [w529 w539]
      tunnel: w386 -> [_ w538]
      tunnel: w383 -> [_ w535]
      tunnel: w376 -> [_ w534]
      tunnel: [w529 w533] -> w381
      tunnel: w374 -> [_ w532]
      tunnel: w373 -> [_ w531]
      frame False {
      }
      frame True {
        n174 = for {
          N: w535 -> [_]
          tunnel: w539 -> [w556]
          tunnel: w538 -> [w569]
          tunnel: w537 -> [w554]
          tunnel: [w558] -> w536
          tunnel: w534 -> [w568]
          tunnel: [w556] -> w533
          tunnel: w532 -> [w550]
          tunnel: w531 -> [w549]
          i -> [w557]
          # "最后两行是电流"
          n175 = Index Array(array=w569, index (row) #1=0 ("禁用的索引 (列)"), index (row) #2=1 ("索引 (列)"), index (row) #3=2 ("索引 (列)")) -> (element #1=w567:dbl[], element #2=w563:dbl[], element #3=w562:dbl[])  [unwired: 3 in]
          n176 = Index Array(array=w554, index (row) #1=w550, index (col) #1=w557, index (row) #2=w549, index (col) #2=w557) -> (element #1=w544:dbl, element #2=w542:dbl)
          n177 = Index Array(array=w556, index (row)=w557, index (col)=w568) -> (element=w553:dbl)
          n178 = Round Toward +Infinity(x=w553) -> (ceil(x): smallest int >= x=w552:dbl)
          n179 = Search 1D Array ("搜索一维数组")(1D array=w567, element=w552) -> (index of element=w564:i32)  [unwired: 1 in]
          n180 = Subtract(x=w552, y=w553) -> (x-y=w551:dbl)
          n181 = Less?(x=w564, y=0) -> (x < y?=w565:bool)
          n182 = case shown="False" w565 {
            tunnel: w564 -> [w582 _]
            tunnel: w563 -> [w584 _]
            tunnel: w562 -> [w583 _]
            tunnel: [w576 1.0] -> w555
            tunnel: [w572 1.0] -> w561
            tunnel: w551 -> [w573 _]
            frame False {
              n183 = Increment(x=w582) -> (x+1=w581:i32)
              n184 = Index Array(array=w583, index #1=w582, index #2=w581) -> (element #1=w570:dbl, element #2=w575:dbl)
              n185 = Index Array(array=w584, index #1=w582, index #2=w581) -> (element #1=w578:dbl, element #2=w580:dbl)
              n186 = Subtract(x=w578, y=w580) -> (x-y=w579:dbl)
              n187 = Subtract(x=w570, y=w575) -> (x-y=w574:dbl)
              n188 = Multiply(x=w579, y=w573) -> (x*y=w577:dbl)
              n189 = Multiply(x=w574, y=w573) -> (x*y=w571:dbl)
              n190 = Subtract(x=w578, y=w577) -> (x-y=w576:dbl)
              n191 = Subtract(x=w570, y=w571) -> (x-y=w572:dbl)
            }
            frame True {
              n192 = One Button Dialog(message="SSF文件棒位索引错误！" ("消息")) -> (true=w588:bool)  [unwired: 1 in]
              n193 = Stop(stop? (T)=w588) -> ()
            }
          }
          n194 = Subtract(x=w542, y="下段本底") -> (x-y=w543:dbl)
          n195 = Subtract(x=w544, y="上段本底") -> (x-y=w545:dbl)
          n196 = Divide(x=w545, y=w555) -> (x/y=w560:dbl)
          n197 = Divide(x=w543, y=w561) -> (x/y=w559:dbl)
          n198 = Replace Array Subset(array=w554, new element #1=w560, index (row) #1=w550, index (col) #1=w557, new element #2=w559, index (row) #2=w549, index (col) #2=w557) -> (w558:dbl[][])
        }
      }
    }
    n199 = Index Array(array=w369, index (col)=0 ("索引 (行)")) -> (element=w366:dbl[])  [unwired: 1 in]
    n200 = Index Array(array=w368, index (col)=0 ("索引 (行)")) -> (element=w367:dbl[])  [unwired: 1 in]
    n201 = global write "GlobalVariable.vi" "Simulate电流"(w366) -> ()
    n202 = global write "GlobalVariable.vi" "Simulate电压"(w367) -> ()
    n203 = Greater?(x="仿真加速或减速倍数", y=1.0) -> (0:w414:bool)
    n204 = case shown="False" w414 {
      tunnel: "仿真加速或减速倍数" -> [w626 w636]
      tunnel: [w627 w635] -> w412
      frame False {
        n205 = Less?(x=w626, y=-1.0) -> (x < y?=w628:bool)
        n206 = case shown="True" w628 {
          tunnel: [1000.0 w633] -> w627
          tunnel: w626 -> [_ w631]
          frame False {
          }
          frame True {
            n207 = Absolute Value(x=w631) -> (abs(x)=w632:dbl)
            n208 = Multiply(x=w632, y=1000.0) -> (x*y=w633:dbl)
          }
        }
      }
      frame True {
        n209 = Divide(x=u32 1000, y=w636) -> (x/y=w635:dbl)
      }
    }
    n210 = And(x="DRWM启用", y="合并DSF") -> (x .and. y?=w371:bool)
    n211 = while {
      tunnel: w389 -> [w641]
      tunnel: [w641] -> w380
      tunnel: w412 -> [w639]
      stop <- w638 stop-if-true
      n212 = Wait (ms)(milliseconds to wait=w639) -> (millisecond timer value=w640:u32)
      n213 = Greater Or Equal?(x=w640, y=w639) -> (x >= y?=w638:bool)
    }
    n214 = case shown="False" w371 {
      tunnel: w380 -> [w457 w470]
      tunnel: [w457 w469] -> w379
      tunnel: w374 -> [w456 w462]
      tunnel: w373 -> [w455 w463]
      frame False {
        n215 = Index Array(array=w457, index (row) #1=w456, index (row) #2=w455) -> (element #1=w461:dbl[], element #2=w460:dbl[])  [unwired: 2 in]
        n216 = Divide(x=w461, y=w460) -> (x/y=w459:dbl[])
        n217 = call-poly <vilib>:"Mean.vi"("X"=w459) -> ("mean"=→"上下段比值":dbl)  [unwired: 1 out]
      }
      frame True {
        n218 = local read "上下段比值"() -> (w467:dbl)
        n219 = Index Array(array=w470, index (row) #1=w462, index (row) #2=w463) -> (element #1=w468:dbl[], element #2=w465:dbl[])  [unwired: 2 in]
        n220 = Divide(x=w468, y=w467) -> (x/y=w466:dbl[])
        n221 = Add(x=w466, y=w465) -> (x+y=w464:dbl[])
        n222 = Replace Array Subset(array=w470, new element #1=w464, index (row) #1=w462, new element #2=w464, index (row) #2=w463) -> (w469:dbl[][])  [unwired: 2 in]
      }
    }
    n223 = call "反应性模拟计算.vi"("循环次数"=w377, "λi*Ci(0)"=w431, "N(0)IN"=w392, "βi"=w432, "λi"=w437, "中子寿命"=w429, "源项"=w428, "采集间隔"=w398, "中子注量率"=w379) -> ("λi*Ci(t)"=w430:sgl[][], "反应性OUT"=w388:sgl[][], "N(0)OUT"=w391:sgl[])  [unwired: 4 in]
    n224 = case shown="True" "DRWM启用" {
      tunnel: w388 -> [w472 w478]
      tunnel: [w472 w481] -> w387
      tunnel: w385 -> [_ w482]
      tunnel: w376 -> [_ w483]
      tunnel: w381 -> [w471 w480]
      tunnel: [w471 w479] -> w384
      tunnel: w374 -> [_ w474]
      tunnel: w373 -> [_ w473]
      frame False {
      }
      frame True {
        n225 = Array Size(array=w478) -> (size(s)=w477:i32[])
        n226 = Index Array(array=w477, index=1 ("索引")) -> (element=w475:i32)
        n227 = for {
          N: w475 -> [_]
          tunnel: w480 -> [w492]
          tunnel: w482 -> [w509]
          tunnel: w478 -> [w497]
          tunnel: [w494] -> w481
          tunnel: w483 -> [w508]
          tunnel: [w492] -> w479
          tunnel: w474 -> [w488]
          tunnel: w473 -> [w487]
          i -> [w493]
          # "最后两行是电流反应性"
          n228 = Index Array(array=w509, index (row) #1=0 ("禁用的索引 (列)"), index (row) #2=1 ("索引 (列)"), index (row) #3=2 ("索引 (列)")) -> (element #1=w507:dbl[], element #2=w503:dbl[], element #3=w502:dbl[])  [unwired: 3 in]
          n229 = Index Array(array=w492, index (row)=w493, index (col)=w508) -> (element=w490:dbl)
          n230 = Round Toward +Infinity(x=w490) -> (ceil(x): smallest int >= x=w491:dbl)
          n231 = Search 1D Array(1D array=w507, element=w491) -> (index of element=w504:i32)  [unwired: 1 in]
          n232 = Index Array(array=w497, index (row) #1=w488, index (col) #1=w493, index (row) #2=w487, index (col) #2=w493) -> (element #1=w501:sgl, element #2=w500:sgl)
          n233 = Subtract(x=w491, y=w490) -> (x-y=w489:dbl)
          n234 = Less?(x=w504, y=0) -> (x < y?=w505:bool)
          n235 = case shown="False" w505 {
            tunnel: w504 -> [w521 _]
            tunnel: w503 -> [w524 _]
            tunnel: w502 -> [w523 _]
            tunnel: [w511 1.0] -> w499
            tunnel: [w510 1.0] -> w498
            tunnel: w489 -> [w516 _]
            frame False {
              n236 = Increment(x=w521) -> (x+1=w522:i32)
              n237 = Index Array(array=w523, index #1=w521, index #2=w522) -> (element #1=w513:dbl, element #2=w519:dbl)
              n238 = Index Array(array=w524, index #1=w521, index #2=w522) -> (element #1=w514:dbl, element #2=w520:dbl)
              n239 = Subtract(x=w514, y=w520) -> (x-y=w518:dbl)
              n240 = Subtract(x=w513, y=w519) -> (x-y=w517:dbl)
              n241 = Multiply(x=w518, y=w516) -> (x*y=w515:dbl)
              n242 = Multiply(x=w517, y=w516) -> (x*y=w512:dbl)
              n243 = Subtract(x=w514, y=w515) -> (x-y=w511:dbl)
              n244 = Subtract(x=w513, y=w512) -> (x-y=w510:dbl)
            }
            frame True {
              n245 = One Button Dialog(message="SSF文件棒位索引错误！" ("消息")) -> (true=w528:bool)  [unwired: 1 in]
              n246 = Stop(stop? (T)=w528) -> ()
            }
          }
          n247 = Multiply(x=w501, y=w499) -> (x*y=w496:dbl)
          n248 = Multiply(x=w500, y=w498) -> (x*y=w495:dbl)
          n249 = Replace Array Subset(array=w497, new element #1=w496, index (row) #1=w488, index (col) #1=w493, new element #2=w495, index (row) #2=w487, index (col) #2=w493) -> (w494:sgl[][])
        }
      }
    }
    n250 = for {
      tunnel: w379 -> [w644] mode=indexing
      tunnel: w387 -> [w643] mode=indexing
      shift-right: [w645] -> w408
      shift-left: sgl[][] [] ("平滑掉数据") -> [w646]
      # "交插通量与反应性"
      n251 = Build Array(w644, w643) -> (w642:dbl[][])
      n252 = Insert Into Array(array=w646, new element=w642) -> (w645:sgl[][])  [unwired: 2 in]
    }
    n253 = Insert Into Array(array=w408, new element=w384) -> (w362:sgl[][])  [unwired: 2 in]
    n254 = Array Size(array=w362) -> (size(s)=w402:i32[])
    n255 = Index Array(array=w402, index=1 ("索引")) -> (element=w400:i32)
    n256 = stacked-sequence {
      tunnel: w375 -> [w447]
      frame #0 {
        # "先后关联不同才能刷新游标图例名！"
        n257 = Array Size(array=w447) -> (size(s)=w446:i32)
        n258 = property on="历史波形图" class="WFGraph (strict)"() -> (error out=w452:errorcluster, "Selected Cursors"=w454:u32[])  [unwired: 2 in, 1 out]
        n259 = Decrement(x=w446) -> (x-1=w441:i32)
        n260 = Index Array(array=w454) -> (element=w453:u32)  [unwired: 1 in]
        n261 = property on="历史波形图" class="WFGraph (strict)"(error in=w452, "Active Cursor"=w453) -> (error out=w451:errorcluster)  [unwired: 1 in, 1 out]
        n262 = property on="历史波形图" class="WFGraph (strict)"(error in=w451) -> (error out=w448:errorcluster, "Cursor.Cursor Plot"=w439:i32)  [unwired: 1 in, 1 out]
        n263 = Increment(x=w439) -> (x+1=w443:i32)
        n264 = Greater Or Equal?(x=w439, y=w441) -> (x >= y?=w450:bool)
        n265 = Greater?(x=w439, y=w441) -> (0:w442:bool)
        n266 = Select(t=0, s=w450, f=w443) -> (s? t:f=w445:i32)
        n267 = Select(t=0, s=w442, f=w439) -> (s? t:f=w440:i32)
        n268 = property on="历史波形图" class="WFGraph (strict)"(error in=w448, "Cursor.Cursor Plot"=w445) -> (error out=w449:errorcluster)  [unwired: 1 in, 1 out]
        n269 = property on="历史波形图" class="WFGraph (strict)"(error in=w449, "Cursor.Cursor Plot"=w440) -> ()  [unwired: 1 in, 2 out]
      }
    }
    n270 = Not Equal?(x="", y="备注说明") -> (x != y?=w406:bool)
    n271 = Transpose 2D Array(2D array=w362) -> (transposed array=→"实时波形图":sgl[][])
    n272 = for {
      N: w400 -> [_]
      tunnel: w394 -> [w594]
      tunnel: w398 -> [w596]
      shift-right: [w592] -> w397
      shift-left: sgl[] [] -> [w593]
      tunnel: [w591] -> w395
      i -> [w590]
      n273 = Increment(x=w590) -> (x+1=w589:i32)
      n274 = Multiply(x=w596, y=w589) -> (x*y=w595:dbl)
      n275 = Add(x=w594, y=w595) -> (x+y=w591:dbl)
      n276 = Insert Into Array(array=w593, new element=w591) -> (w592:sgl[])  [unwired: 1 in]
    }
    n277 = Insert Into Array ("数组插入")(array=w362, index (row)=0 ("索引 (行)"), new element=w397) -> (w396:sgl[][])  [unwired: 1 in]
    n278 = Transpose 2D Array(2D array=w396) -> (transposed array=w424:sgl[][])
    n279 = Array To Spreadsheet String(array=w424, 3:"%g" ("format string")) -> (spreadsheet string=w382:string)  [unwired: 1 in]
    n280 = case shown="True" w406 {
      tunnel: [w597 w598] -> w403
      tunnel: "备注说明" -> [_ w607]
      tunnel: w382 -> [w597 w602]
      frame False {
      }
      frame True {
        n281 = Spreadsheet String To Array(delimiter (Tab)="\t", format string="%s", spreadsheet string=w602, array type (2D Dbl)=string[][] [] ("添加的数组")) -> (array=w603:string[][])
        n282 = for {
          tunnel: w603 -> [w617] mode=indexing
          tunnel: [w616] -> w601 mode=indexing
          tunnel: w607 -> [w611]
          i -> [w615]
          n283 = Not Equal?(x=0 ("y"), y=w615) -> (x != y?=w613:bool)
          n284 = Select(t="", s=w613, f=w611) -> (s? t:f=w612:string)
          n285 = Insert Into Array(array=w617, new element=w612) -> (w616:string[])  [unwired: 1 in]
        }
        n286 = flat-sequence {
          tunnel: w601 -> [w608]
          tunnel: [w608] -> w599
          frame #0 {
            n287 = local write "备注说明"("") -> ()
          }
        }
        n288 = Array To Spreadsheet String(array=w599, 3:"%s" ("format string")) -> (spreadsheet string=w598:string)  [unwired: 1 in]
      }
    }
    n289 = Index Array(array=w362, index (col)=0 ("索引 (行)")) -> (element=w421:sgl[])  [unwired: 1 in]
    n290 = Index Array(array=w421) -> (element #1=→"曲线0数字":sgl, element #2=→"曲线1数字":sgl, element #3=→"曲线2数字":sgl, element #4=→"曲线3数字":sgl, element #5=→"曲线4数字":sgl, element #6=→"曲线5数字":sgl)  [unwired: 6 in]
    n291 = local read "数据采集起止时间"() -> (w390:string)
    n292 = Write to Binary File(file (use dialog)=w427, data=w403, error in=w435, 5:FALSE ("预置数组或字符串大小？(T)")) -> (refnum out=w426:refnum<file>, error out=w434:errorcluster)  [unwired: 2 in, 1 out]
    n293 = flat-sequence {
      tunnel: [w619] -> w361
      frame #0 {
        n294 = local read "退出"() -> (w618:bool)
        n295 = local write "AllStop"(w618) -> ()
      }
      frame #1 {
        n296 = local read "AllStop"() -> (w619:bool)
      }
    }
  }
  n297 = while {
    tunnel: w112 -> [w678]
    tunnel: w121 -> [w653]
    tunnel: w120 -> [w652]
    stop <- w692 stop-if-true
    w676 = bool[] []  # 记录有无手动标尺
    # "显隐曲线并集合用到的标尺"
    n298 = property on="AllStop" class="Bool (strict)"() -> ("值"=w692:bool)  [unwired: 2 in, 2 out]
    n299 = call-poly <vilib>:"Acquire Input Data.vi"("device ID"=w652, "error in (no error)"=w653) -> ("button info"=w654:T5)  [unwired: 1 in, 16 out]
    n300 = Unbundle By Name(w654) -> ("button 1"=w651:bool, "button 2"=w650:bool, "button 3"=w649:bool, "button 4"=w648:bool)
    n301 = property on="X标尺最小-" class="Bool"("Visible"="自动/手动调整X标尺？") -> ()  [unwired: 2 in, 2 out]
    n302 = property on="X标尺最小+" class="Bool"("Visible"="自动/手动调整X标尺？") -> (error out=w670:errorcluster)  [unwired: 2 in, 1 out]
    n303 = Build Array("曲线开关0", "曲线开关1", "曲线开关2", "曲线开关3", "曲线开关4", "曲线开关5") -> (w685:bool[])
    n304 = Compound Arithmetic op=OR(w651, w650, w649, w648) -> (w647:bool)
    n305 = property on="实时波形图" class="WFChart (strict)"() -> (error out=w679:errorcluster, "History Data"=w668:sgl[][])  [unwired: 2 in, 1 out]
    n306 = case shown="False" w647 {
      frame False {
        n307 = Wait Until Next ms Multiple(millisecond multiple=u32 1000) -> ()  [unwired: 1 out]
      }
      frame True {
        n308 = Wait Until Next ms Multiple(millisecond multiple=u32 100) -> ()  [unwired: 1 out]
      }
    }
    n309 = Array Size(array=w668) -> (size(s)=w667:i32[])
    n310 = property on="实时波形图" class="WFChart (strict)"(error in=w670, "ActXScl"=0 ("活动X标尺")) -> (error out=w664:errorcluster)  [unwired: 1 in, 1 out]
    n311 = for {
      tunnel: w685 -> [w915] mode=indexing
      tunnel: w678 -> [w913] mode=indexing
      shift-right: [w912] -> w682
      shift-left: i32[] [] ("添加的数组") -> [w914]
      shift-right: [w909] -> w680
      shift-left: i32[] [] ("添加的数组") -> [w911]
      i -> [w910]
      n312 = property on="实时波形图" class="WFChart (strict)"("活动曲线"=w910, "曲线.可见"=w915) -> ()  [unwired: 2 in, 2 out]
      n313 = case shown="False" w915 {
        tunnel: w914 -> [w917 w923]
        tunnel: w913 -> [_ w922]
        tunnel: [w917 w921] -> w912
        tunnel: w911 -> [w916 w920]
        tunnel: w910 -> [_ w919]
        tunnel: [w916 w918] -> w909
        frame False {
        }
        frame True {
          n314 = Insert Into Array(array=w920, new element=w919) -> (w918:i32[])  [unwired: 1 in]
          n315 = Insert Into Array(array=w923, new element=w922) -> (w921:i32[])  [unwired: 1 in]
        }
      }
    }
    n316 = Index Array(array=w667, index=1 ("索引")) -> (element=w665:i32)
    n317 = property on="实时波形图" class="WFChart (strict)"(error in=w664) -> (error out=w663:errorcluster, "XScale.Maximum"=w661:dbl)  [unwired: 1 in, 1 out]
    n318 = for {
      N: 8 -> [_]
      tunnel: w682 -> [w752]
      tunnel: w680 -> [w753]
      tunnel: w679 -> [w751]
      tunnel: w668 -> [w750]
      tunnel: "自动调整Y标尺？" -> [w748]
      shift-right: [w746] -> w675
      shift-left: w676 -> [w747]
      i -> [w754]
      # "根据标尺有无被用到决定是否显示标尺"
      n319 = for {
        tunnel: w752 -> [w908] mode=indexing
        tunnel: w754 -> [w907]
        tunnel: [w906] -> w755
        stop <- w906 stop-if-true
        n320 = Equal?(x=w908, y=w907) -> (x = y?=w906:bool)
      }
      n321 = property on="实时波形图" class="WFChart (strict)"("ActYScl"=w754) -> (error out=w756:errorcluster)  [unwired: 2 in, 1 out]
      n322 = property on="实时波形图" class="WFChart (strict)"(error in=w756, "YScale.Visible"=w755) -> (error out=w749:errorcluster)  [unwired: 1 in, 1 out]
      n323 = case shown="True" w755 {
        tunnel: w754 -> [_ w776]
        tunnel: w753 -> [_ w775]
        tunnel: w752 -> [_ w777]
        tunnel: w751 -> [_ w774]
        tunnel: w750 -> [_ w773]
        tunnel: w749 -> [_ w765]
        tunnel: w748 -> [_ w763]
        tunnel: w747 -> [w757 w760]
        tunnel: [w757 w759] -> w746
        frame False {
        }
        frame True {
          n324 = property on="实时波形图" class="WFChart (strict)"(error in=w765) -> ("YScale.Increment"=w764:dbl)  [unwired: 1 in, 2 out]
          n325 = property on="实时波形图" class="WFChart (strict)"(error in=w765) -> (error out=w767:errorcluster, "YScale.ScaleFit"=w770:u8)  [unwired: 1 in, 1 out]
          n326 = for {
            tunnel: w777 -> [w886] mode=indexing
            tunnel: w776 -> [w885]
            tunnel: w775 -> [w884]
            tunnel: w774 -> [w881]
            tunnel: w773 -> [w880]
            shift-right: [w877] -> w766
            shift-left: inf -> [w879]
            shift-right: [w876] -> w768
            shift-left: -inf -> [w878]
            i -> [w883]
            # "正在显示的标尺则考虑调整"
            n327 = Equal?(x=w886, y=w885) -> (x = y?=w882:bool)
            n328 = case shown="True" w882 {
              tunnel: w884 -> [_ w901]
              tunnel: w883 -> [_ w900]
              tunnel: w881 -> [_ _]
              tunnel: w880 -> [_ w899]
              tunnel: [w888 w892] -> w877
              tunnel: w879 -> [w888 w891]
              tunnel: w878 -> [w887 w895]
              tunnel: [w887 w894] -> w876
              frame False {
              }
              frame True {
                n329 = Index Array(array=w901, index=w900) -> (element=w898:i32)
                n330 = Index Array(array=w899, index (row)=w898) -> (element=w897:sgl[])  [unwired: 1 in]
                n331 = Array Max & Min(array=w897) -> (max value=w893:sgl, min value=w890:sgl)  [unwired: 2 out]
                n332 = Greater?(x=w893, y=w895) -> (0:w896:bool)
                n333 = Less?(x=w890, y=w891) -> (x < y?=w889:bool)
                n334 = case shown="True" w896 {
                  tunnel: w895 -> [w904 _]
                  tunnel: [w904 w905] -> w894
                  tunnel: w893 -> [_ w905]
                  frame False {
                  }
                  frame True {
                  }
                }
                n335 = case shown="True" w889 {
                  tunnel: w891 -> [w902 _]
                  tunnel: [w902 w903] -> w892
                  tunnel: w890 -> [_ w903]
                  frame False {
                  }
                  frame True {
                  }
                }
              }
            }
          }
          n336 = Equal?(x=w770, y=u8 0) -> (x = y?=w761:bool)
          n337 = case shown="True" w761 {
            selector: w761 -> [w793 _]
            tunnel: w768 -> [_ w804]
            tunnel: w767 -> [w792 w815]
            tunnel: w766 -> [_ w799]
            tunnel: w761 -> [_ _]
            tunnel: w764 -> [_ w796]
            tunnel: [w792 w795] -> w762
            tunnel: [w793 w794] -> w758
            tunnel: w761 -> [_ w794]
            frame False {
            }
            frame True {
              n338 = property on="实时波形图" class="WFChart (strict)"(error in=w815) -> (error out=w813:errorcluster, "YScale.Maximum"=w814:dbl)  [unwired: 1 in, 1 out]
              n339 = property on="实时波形图" class="WFChart (strict)"(error in=w815) -> (error out=w805:errorcluster, "YScale.Minimum"=w806:dbl)  [unwired: 1 in, 1 out]
              n340 = case shown="True" "Y标尺最小+" {
                tunnel: w804 -> [_ w839]
                tunnel: w806 -> [w831 w837]
                tunnel: w805 -> [w832 w836]
                tunnel: [w832 w835] -> w802
                tunnel: [w831 w834] -> w800
                tunnel: w796 -> [_ w833]
                frame False {
                }
                frame True {
                  n341 = Greater?(x=w837, y=w839) -> (0:w838:bool)
                  n342 = case shown="False" w838 {
                    tunnel: [w841 w845] -> w834
                    tunnel: w839 -> [_ w845]
                    tunnel: w837 -> [w842 _]
                    tunnel: w836 -> [w843 w844]
                    tunnel: [w843 w844] -> w835
                    tunnel: w833 -> [w840 _]
                    frame False {
                      n343 = Add(x=w842, y=w840) -> (x+y=w841:dbl)
                    }
                    frame True {
                    }
                  }
                }
              }
              n344 = case shown="True" "Y标尺最大+" {
                tunnel: w804 -> [_ w869]
                tunnel: w814 -> [w861 w867]
                tunnel: w813 -> [w862 w866]
                tunnel: [w862 w865] -> w810
                tunnel: [w861 w864] -> w809
                tunnel: w796 -> [_ w863]
                frame False {
                }
                frame True {
                  n345 = Greater?(x=w867, y=w869) -> (0:w868:bool)
                  n346 = case shown="False" w868 {
                    tunnel: [w871 w875] -> w864
                    tunnel: w869 -> [_ w875]
                    tunnel: w867 -> [w872 _]
                    tunnel: w866 -> [w873 w874]
                    tunnel: [w873 w874] -> w865
                    tunnel: w863 -> [w870 _]
                    frame False {
                      n347 = Add(x=w872, y=w870) -> (x+y=w871:dbl)
                    }
                    frame True {
                    }
                  }
                }
              }
              n348 = case shown="True" "Y标尺最大-" {
                tunnel: w799 -> [_ w854]
                tunnel: w809 -> [w847 w852]
                tunnel: w810 -> [w846 w851]
                tunnel: [w847 w850] -> w808
                tunnel: [w846 w849] -> w807
                tunnel: w796 -> [_ w848]
                frame False {
                }
                frame True {
                  n349 = Less?(x=w852, y=w854) -> (x < y?=w853:bool)
                  n350 = case shown="False" w853 {
                    tunnel: [w856 w860] -> w850
                    tunnel: w854 -> [_ w860]
                    tunnel: w852 -> [w857 _]
                    tunnel: w851 -> [w858 w859]
                    tunnel: [w858 w859] -> w849
                    tunnel: w848 -> [w855 _]
                    frame False {
                      n351 = Subtract(x=w857, y=w855) -> (x-y=w856:dbl)
                    }
                    frame True {
                    }
                  }
                }
              }
              n352 = case shown="True" "Y标尺最小-" {
                tunnel: w799 -> [_ w824]
                tunnel: w800 -> [w817 w822]
                tunnel: w802 -> [w816 w821]
                tunnel: [w817 w820] -> w797
                tunnel: [w816 w819] -> w798
                tunnel: w796 -> [_ w818]
                frame False {
                }
                frame True {
                  n353 = Less?(x=w822, y=w824) -> (x < y?=w823:bool)
                  n354 = case shown="False" w823 {
                    tunnel: [w826 w830] -> w820
                    tunnel: w824 -> [_ w830]
                    tunnel: w822 -> [w827 _]
                    tunnel: w821 -> [w828 w829]
                    tunnel: [w828 w829] -> w819
                    tunnel: w818 -> [w825 _]
                    frame False {
                      n355 = Subtract(x=w827, y=w825) -> (x-y=w826:dbl)
                    }
                    frame True {
                    }
                  }
                }
              }
              n356 = property on="实时波形图" class="WFChart (strict)"(error in=w807, "YScale.Maximum"=w808) -> (error out=w795:errorcluster)  [unwired: 1 in, 1 out]
              n357 = property on="实时波形图" class="WFChart (strict)"(error in=w798, "YScale.Minimum"=w797) -> ()  [unwired: 1 in, 2 out]
            }
          }
          n358 = case shown="True" w763 {
            tunnel: w762 -> [_ w783]
            tunnel: w758 -> [_ w781]
            frame False {
            }
            frame True {
              n359 = property on="实时波形图" class="WFChart (strict)"(error in=w783) -> (error out=w780:errorcluster, "YScale.NameLbl.Text"=w785:string)  [unwired: 1 in, 1 out]
              n360 = Select(t="-手动调整转为自动调整？" ("format string"), s=w781, f="-自动调整转为手动调整？" ("format string")) -> (s? t:f=w786:string)
              n361 = Concatenate Strings ("连接字符串")(w785, w786) -> (w784:string)
              n362 = call "Dialog_Box.vi"("提示信息"=w784) -> ("选择结果"=w782:bool)
              n363 = case shown="True" w782 {
                tunnel: w781 -> [_ w791]
                tunnel: w780 -> [_ w787]
                frame False {
                }
                frame True {
                  n364 = Select(t=u8 2 ("y"), s=w791, f=u8 0 ("y")) -> (s? t:f=w788:u8)
                  n365 = property on="实时波形图" class="WFChart (strict)"(error in=w787, "YScale.ScaleFit"=w788) -> ()  [unwired: 1 in, 2 out]
                }
              }
            }
          }
          n366 = Insert Into Array(array=w760, new element=w758) -> (w759:bool[])  [unwired: 1 in]
        }
      }
    }
    n367 = property on="实时波形图" class="WFChart (strict)"(error in=w663) -> (error out=w662:errorcluster, "XScale.Minimum"=w660:dbl)  [unwired: 1 in, 1 out]
    n368 = Subtract(x=w661, y=w660) -> (x-y=w659:dbl)
    n369 = Multiply(x=w659, y=0.1) -> (x*y=w657:dbl)
    n370 = Round Toward +Infinity(x=w657) -> (ceil(x): smallest int >= x=w656:dbl)
    n371 = case shown="True" "自动/手动调整X标尺？" {
      tunnel: [2 ("活动X标尺") 0 ("活动X标尺")] -> w671
      tunnel: [w717 w719] -> w669
      tunnel: w662 -> [w717 w730]
      tunnel: w665 -> [_ w735]
      tunnel: w660 -> [_ w729]
      tunnel: w656 -> [_ w721]
      frame False {
      }
      frame True {
        n372 = Subtract(x=w735, y=10.0) -> (x-y=w728:dbl)
        n373 = Subtract(x=w728, y=w721) -> (x-y=w727:dbl)
        n374 = Less?(x=w729, y=w727) -> (x < y?=w732:bool)
        n375 = And(x="X标尺最小+", y=w732) -> (x .and. y?=w734:bool)
        n376 = case shown="True" w734 {
          tunnel: w729 -> [w742 w745]
          tunnel: [w742 w744] -> w723
          tunnel: w721 -> [_ w743]
          frame False {
          }
          frame True {
            n377 = Add(x=w745, y=w743) -> (x+y=w744:dbl)
          }
        }
        n378 = Add(x=10.0, y=w721) -> (x+y=w720:dbl)
        n379 = Greater?(x=w723, y=w720) -> (0:w724:bool)
        n380 = And(x="X标尺最小-", y=w724) -> (x .and. y?=w726:bool)
        n381 = case shown="True" w726 {
          tunnel: w723 -> [w738 w741]
          tunnel: [w738 w740] -> w731
          tunnel: w721 -> [_ w739]
          frame False {
          }
          frame True {
            n382 = Subtract(x=w741, y=w739) -> (x-y=w740:dbl)
          }
        }
        n383 = property on="实时波形图" class="WFChart (strict)"(error in=w730, "XScale.Minimum"=w731) -> (error out=w719:errorcluster)  [unwired: 1 in, 1 out]
      }
    }
    n384 = property on="实时波形图" class="WFChart (strict)"(error in=w669, "XScale.ScaleFit"=w671) -> ()  [unwired: 1 in, 2 out]
    n385 = for {
      N: 6 -> [_]
      i -> [w695]
      # "数值显示颜色同步于曲线"
      n386 = property on="实时波形图" class="WFChart (strict)"("Active Plot"=w695) -> (error out=w698:errorcluster)  [unwired: 2 in, 1 out]
      n387 = property on="实时波形图" class="WFChart (strict)"(error in=w698) -> (error out=w697:errorcluster, "Plot.Plot Color"=w696:u32)  [unwired: 1 in, 1 out]
      n388 = case shown="5" w695 {
        tunnel: w697 -> [w700 w703 w706 w709 w712 w715]
        tunnel: w696 -> [w699 w702 w705 w708 w711 w714]
        frame 1 {
          n389 = property on="曲线1数字" class="DigNum (strict)"(error in=w700, "Caption.TextColor"=w699) -> (error out=w701:errorcluster)  [unwired: 1 in, 1 out]
          n390 = property on="曲线1数字" class="DigNum (strict)"(error in=w701, "NumText.TextColor"=w699) -> ()  [unwired: 1 in, 2 out]
        }
        frame 2 {
          n391 = property on="曲线2数字" class="DigNum (strict)"(error in=w703, "Caption.TextColor"=w702) -> (error out=w704:errorcluster)  [unwired: 1 in, 1 out]
          n392 = property on="曲线2数字" class="DigNum (strict)"(error in=w704, "NumText.TextColor"=w702) -> ()  [unwired: 1 in, 2 out]
        }
        frame 3 {
          n393 = property on="曲线3数字" class="DigNum (strict)"(error in=w706, "Caption.TextColor"=w705) -> (error out=w707:errorcluster)  [unwired: 1 in, 1 out]
          n394 = property on="曲线3数字" class="DigNum (strict)"(error in=w707, "NumText.TextColor"=w705) -> ()  [unwired: 1 in, 2 out]
        }
        frame 4 {
          n395 = property on="曲线4数字" class="DigNum (strict)"(error in=w709, "Caption.TextColor"=w708) -> (error out=w710:errorcluster)  [unwired: 1 in, 1 out]
          n396 = property on="曲线4数字" class="DigNum (strict)"(error in=w710, "NumText.TextColor"=w708) -> ()  [unwired: 1 in, 2 out]
        }
        frame 5 {
          n397 = property on="曲线5数字" class="DigNum (strict)"(error in=w712, "Caption.TextColor"=w711) -> (error out=w713:errorcluster)  [unwired: 1 in, 1 out]
          n398 = property on="曲线5数字" class="DigNum (strict)"(error in=w713, "NumText.TextColor"=w711) -> ()  [unwired: 1 in, 2 out]
        }
        frame 0, Default {
          n399 = property on="曲线0数字" class="DigNum (strict)"(error in=w715, "Caption.TextColor"=w714) -> (error out=w716:errorcluster)  [unwired: 1 in, 1 out]
          n400 = property on="曲线0数字" class="DigNum (strict)"(error in=w716, "NumText.TextColor"=w714) -> ()  [unwired: 1 in, 2 out]
        }
      }
    }
    n401 = Or Array Elements(Boolean array=w675) -> (logical OR=w674:bool)
    n402 = property on="Y标尺最小-" class="Bool"("Visible"=w674) -> ()  [unwired: 2 in, 2 out]
    n403 = property on="Y标尺最小+" class="Bool"("Visible"=w674) -> ()  [unwired: 2 in, 2 out]
    n404 = property on="Y标尺最大+" class="Bool"("Visible"=w674) -> ()  [unwired: 2 in, 2 out]
    n405 = property on="Y标尺最大-" class="Bool"("Visible"=w674) -> ()  [unwired: 2 in, 2 out]
  }
  n406 = while {
    stop <- FALSE stop-if-true
    n407 = event shown="[2] \"曲线标尺\": Value Change" {
      selector: _ -> [_ _ _]
      dyn-events: _ -> [_ _ _]
      timeout: _ -> [_ _ _]
      event Timeout {
        n408 = event-data() -> ()  [unwired: 1 in, 3 out]
      }
      event "曲线隐显": Value Change {
        n409 = event-data() -> ("CtlRef"=w926:refnum<vi>)  [unwired: 1 in, 3 out]
        n410 = property class="Arr (strict)"(reference=w926) -> ("Value"=w925:bool[])  [unwired: 1 in, 2 out]
        n411 = for {
          tunnel: w925 -> [w927] mode=indexing
          i -> [w928]
          n412 = property on="历史波形图" class="WFGraph (strict)"("Active Plot"=w928) -> (error out=w929:errorcluster)  [unwired: 2 in, 1 out]
          n413 = property on="历史波形图" class="WFGraph (strict)"(error in=w929, "Plot.Visible?"=w927) -> ()  [unwired: 1 in, 2 out]
        }
      }
      event "曲线标尺": Value Change {
        n414 = event-data() -> ("CtlRef"=w931:refnum<vi>)  [unwired: 1 in]
        n415 = property class="Arr (strict)"(reference=w931) -> ("Value"=w930:bool[])  [unwired: 1 in, 2 out]
        n416 = for {
          tunnel: w930 -> [w933] mode=indexing
          i -> [w934]
          n417 = property on="历史波形图" class="WFGraph (strict)"("ActYScl"=w934) -> (error out=w932:errorcluster)  [unwired: 2 in, 1 out]
          n418 = property on="历史波形图" class="WFGraph (strict)"(error in=w932, "YScale.Visible"=w933) -> ()  [unwired: 1 in, 2 out]
        }
      }
    }
  }
  n419 = flat-sequence {
    tunnel: w113 -> [_]
    frame #0 {
      # "清空曲线区域"
      n420 = local write "退出"(FALSE ("取消")) -> ()
    }
    frame #1 {
      n421 = case shown="True" TRUE {
        frame False {
        }
        frame True {
          n422 = invoke class="VI" method="FP.Close"() -> (reference out=w937:refnum<vi>, error out=w938:errorcluster)  [unwired: 3 in, 1 out]
          n423 = Close Reference(reference=w937, error in (no error)=w938) -> ()  [unwired: 1 out]
        }
      }
    }
  }
  n424 = Write to Binary File(file (use dialog)=w80, data=w74, error in=w79, 5:FALSE ("预置数组或字符串大小？(T)")) -> (refnum out=w82:refnum<file>, error out=w81:errorcluster)  [unwired: 2 in, 1 out]
  n425 = Close File(refnum=w82, error in=w81) -> (error out=w83:errorcluster)  [unwired: 1 out]
  n426 = call <vilib>:"Simple Error Handler.vi"("error in (no error)"=w83) -> ()  [unwired: 4 in, 5 out]
  n427 = property class="Clust (strict)"("Visible"=w5) -> ()  [unwired: 2 in, 2 out]
  n428 = property on="重选文件" class="Bool"("Visible"=w5) -> ()  [unwired: 2 in, 2 out]
